vi "LinxAnalogRead.vi"(8 "Error In":errorcluster, 10 "Channels":u8[](array[numeric]), 11 "LINX Resource":T1) -> (0 "Error Out":errorcluster, 1 "AI Ref":dbl, 2 "AI Values":dbl[](array[numeric]), 3 "LINX Resource":T1)   [LabVIEW 2014, in "LMH-LINX.lvlib" / "Local IO.lvlib"]
uses:
  <vilib>/MakerHub/LINX/Private/Local IO/Local IO.lvlib
  <vilib>/MakerHub/LINX/Private/Type Defs/LINX Ref.ctl
  <vilib>/MakerHub/LINX/Private/Type Defs/Platform.ctl
  <vilib>/MakerHub/LINX/Private/Type Defs/Interface.ctl
  <vilib>/MakerHub/LINX/Private/Device/Type Defs/LINX Device Config.ctl
  <vilib>/MakerHub/LINX/Private/Device/Type Defs/TCP Config.ctl
  <vilib>/MakerHub/LINX/Private/Device/Type Defs/Channels.ctl
  <vilib>/myRIO/Instrument Drivers/Onboard IO/AI/AI.lvlib
  <vilib>/MakerHub/LINX/Private/Type Defs/Error Type.ctl
  <vilib>/MakerHub/LINX/LMH-LINX.lvlib
  <vilib>/MakerHub/LINX/Private/myRIO/myRIO.lvlib
  liblinxdevice.dll
  <vilib>/MakerHub/LINX/Private/Device/Device.lvlib
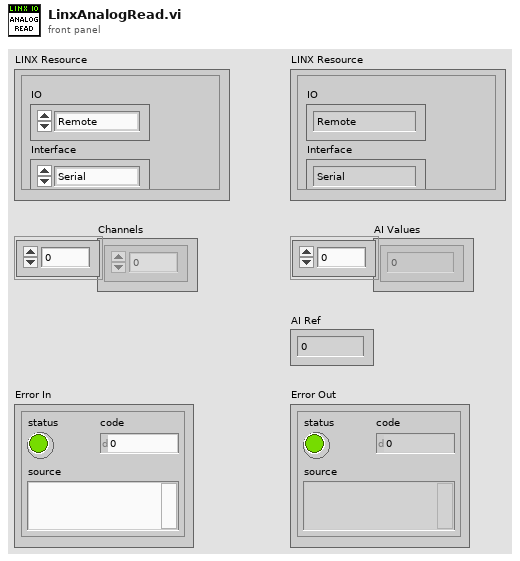
[diagram p1: front panel]
types:
  T1 = typedef "LMH-LINX.lvlib/LINX Ref.ctl" = cluster{"IO":T2, "Interface":T3, "LINX Device Config":T4}
  T2 = typedef "LMH-LINX.lvlib/Platform.ctl" = enum16{"Remote", "Local"}
  T3 = typedef "LMH-LINX.lvlib/Interface.ctl" = enum16{"Serial", "TCP"}
  T4 = typedef "LMH-LINX.lvlib/Device.lvlib/LINX Device Config.ctl" = cluster{"Interface":T3, "COM Port":refnum<visa-resource-name>, "TCP Configuration":T5, "Device Family":u8, "Device ID":u8, "Device Name":string, "TCP Ref":refnum<k5>, "Channels":T6}
  T5 = typedef "LMH-LINX.lvlib/Device.lvlib/TCP Config.ctl" = cluster{"IP Address":string, "Port":u16}
  T6 = typedef "LMH-LINX.lvlib/Channels.ctl" = cluster{"DI":u8[], "DO":u8[], "AI":u8[], "AO":u8[], "PWM":u8[], "QE":u8[], "UART":u8[], "I2C 2":u8[], "SPI":u8[], "CAN":u8[], "Servo":u8[], "AI Ref (V)":dbl, "AI Resolution (Bits)":u8, "AO Ref (V)":dbl, "AO Resolution (Bits)":u8}
  T7 = typedef "LMH-LINX.lvlib/Error Type.ctl" = enum16{"Unknown", "Timeout", "Corrupt Return Packet", "Unable To Connect", "Command Not Supported", "Channel DNE", "Invalid COM Config", "Firmware Version Mismatch", "myRIO Support", "CMD Specific Error", "Local IO Not Supported"}
  T8 = typedef "AI.lvlib/AI Reference.ctl" = cluster{"myRIO Reference":T9, "AI Channels List":T13, "AI Scaling Constants List":T15}
  T9 = typedef "myRIO Generic Hardware Reference.ctl" = cluster{"myRIO Model":T10, "myRIO Hardware Reference":T11}
  T10 = typedef "Hardware Version Enum.ctl" = enum16{"Unknown", "myRIO-1900", "myRIO-1950"}
  T11 = typedef "myRIO v1.0 Reference.ctl" = cluster{"Generic FPGA Reference":T12, "Allow multiple opens":bool}
  T12 = typedef "Generic FPGA Reference.ctl" = refnum<k20>
  T13 = typedef "AI Channels List.ctl" = T14[]
  T14 = typedef "AI Channels Enum.ctl" = enum16{"Not Connected", "AudioIn/Left", "AudioIn/Right", "C/AI0", "C/AI1", "A/AI0", "A/AI1", "A/AI2", "A/AI3", "B/AI0", "B/AI1", "B/AI2", "B/AI3"}
  T15 = typedef "Analog Scaling Constants List.ctl" = T16[]
  T16 = typedef "Analog Scaling Constants.ctl" = cluster{"LSB Weight (Volts)":dbl, "Offset (Volts)":dbl, "Signed?":bool}
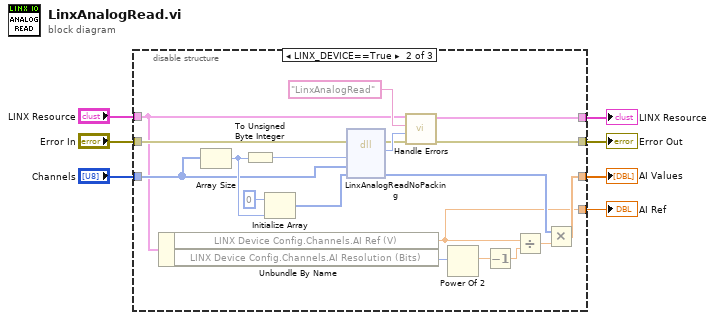
[diagram p0: block diagram]
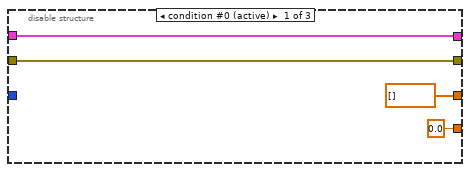
[diagram p2: hidden frame]
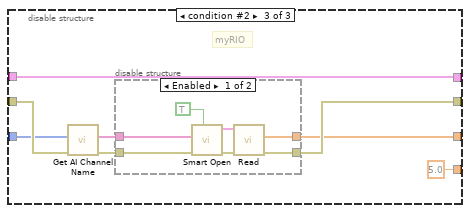
[diagram p3: hidden frame]
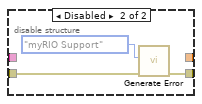
[diagram p4: hidden frame]
diagram:
  n1 = disable-structure shown="LINX_DEVICE==True" {
    disable-tunnel: [w11 w23 w38] -> w7
    disable-tunnel: [w10 w22 w35] -> w6
    disable-tunnel: "LINX Resource" -> [w11 w19 w38]
    disable-tunnel: "Error In" -> [w10 w21 w34]
    disable-tunnel: "Channels" -> [_ w20 w33]
    disable-tunnel: [dbl[] [] ("AI Values") w17 w32] -> w2
    disable-tunnel: [0.0 ("AI Ref") w16 5.0 ("AI Ref")] -> w1
    frame condition #0 (active) {
    }
    frame condition #1 {
      n2 = Unbundle By Name(w19) -> ("LINX Device Config.Channels.AI Ref (V)"=w16:dbl, "LINX Device Config.Channels.AI Resolution (Bits)"=w15:u8)
      n3 = Array Size(array=w20) -> (size(s)=w25:i32)
      n4 = To Unsigned Byte Integer(number=w25) -> (unsigned 8bit integer=w24:u8)
      n5 = Initialize Array(u32 0 ("element"), w25) -> (w30:u32[])
      n6 = dll-call lib="liblinxdevice.*" fn="LinxAnalogReadNoPacking"(error in=w21, "numChans"=w24, "channels"=w20, "values"=w30) -> (error out=w26:errorcluster, "LinxStatus"=w27:i32, "values"=w18:u32[])  [unwired: 4 in, 1 out]
      n7 = call <vilib>:"Handle Errors.vi"("Error In"=w26, "LinxStatus"=w27, "Function Name"="LinxAnalogRead", "LINX Resource"=w19) -> ("Error Out"=w22:errorcluster, "LINX Resource"=w23:T1)  [unwired: 6 in]
      n8 = Power Of 2(x=w15) -> (2^x=w12:dbl)
      n9 = Decrement(x=w12) -> (x-1=w14:dbl)
      n10 = Divide(x=w16, y=w14) -> (x/y=w13:dbl)
      n11 = Multiply(x=w18, y=w13) -> (x*y=w17:dbl[])
    }
    frame condition #2 {
      # "myRIO"
      n12 = call <vilib>:"Get AI Channel Name.vi"("Error In"=w34, "AI Channel Nums"=w33) -> ("Error Out"=w36:errorcluster, "AI Channels"=w37:string[])  [unwired: 7 in]
      n13 = disable-structure shown="Enabled" {
        disable-tunnel: w36 -> [w43 w48]
        disable-tunnel: [w42 w47] -> w35
        disable-tunnel: w37 -> [w40 _]
        disable-tunnel: [w39 _] -> w32
        frame Enabled {
          n14 = call <vilib>:"Smart Open.vi"("Allow multiple opens?"=TRUE, "error in (no error)"=w43, "Channel Names"=w40) -> ("error out"=w45:errorcluster, "AI Ref Out"=w44:T8)  [unwired: 7 in]
          n15 = call <vilib>:"Read.vi"("error in (no error)"=w45, "AI Ref In"=w44) -> ("error out"=w42:errorcluster, "Values"=w39:dbl[])  [unwired: 7 in, 1 out]
        }
        frame Disabled {
          n16 = call <vilib>:"Generate Error.vi"("Error In"=w48, "Error Type"=Error_Type."myRIO Support") -> ("Error Out"=w47:errorcluster)  [unwired: 8 in, 1 out]
        }
      }
    }
  }
  "Error Out" <- w6
  "LINX Resource" <- w7
  "AI Values" <- w2
  "AI Ref" <- w1
